vi "PRM1Z8_Init.vi"(8 "error in (no error)":errorcluster) -> (0 "error out":errorcluster, 3 "reference out":refnum<k24>)   [LabVIEW 2023, in "Thorlabs Polarizer.lvlib"]
uses:
  C:/FlashGordon/Development/dll/ThorLabs.MotionControl.KCube.DCServoCLI.dll
  dll/ThorLabs.MotionControl.KCube.DCServoCLI.dll
  C:/FlashGordon/Development/dll/Thorlabs.MotionControl.DeviceManagerCLI.dll
  dll/Thorlabs.MotionControl.DeviceManagerCLI.dll
  C:/FlashGordon/Development/dll/Thorlabs.MotionControl.GenericMotorCLI.dll
  dll/Thorlabs.MotionControl.GenericMotorCLI.dll
  Thorlabs Polarizer.lvlib
panel:
  out "Controller Information":T1
  out "Device list (serial no.)":string[](array[string])
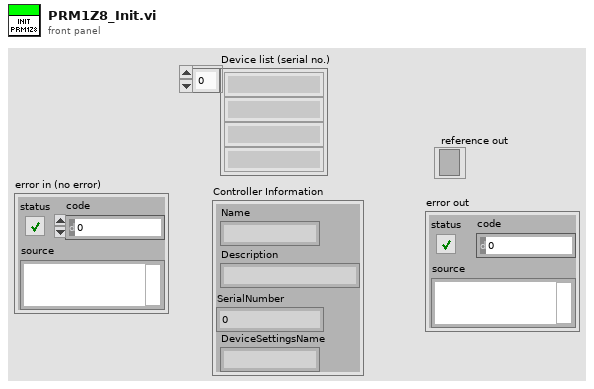
[diagram p1: front panel]
types:
  T1 = cluster{"Name":string, "Description":string, "SerialNumber":u32, "DeviceSettingsName":string}
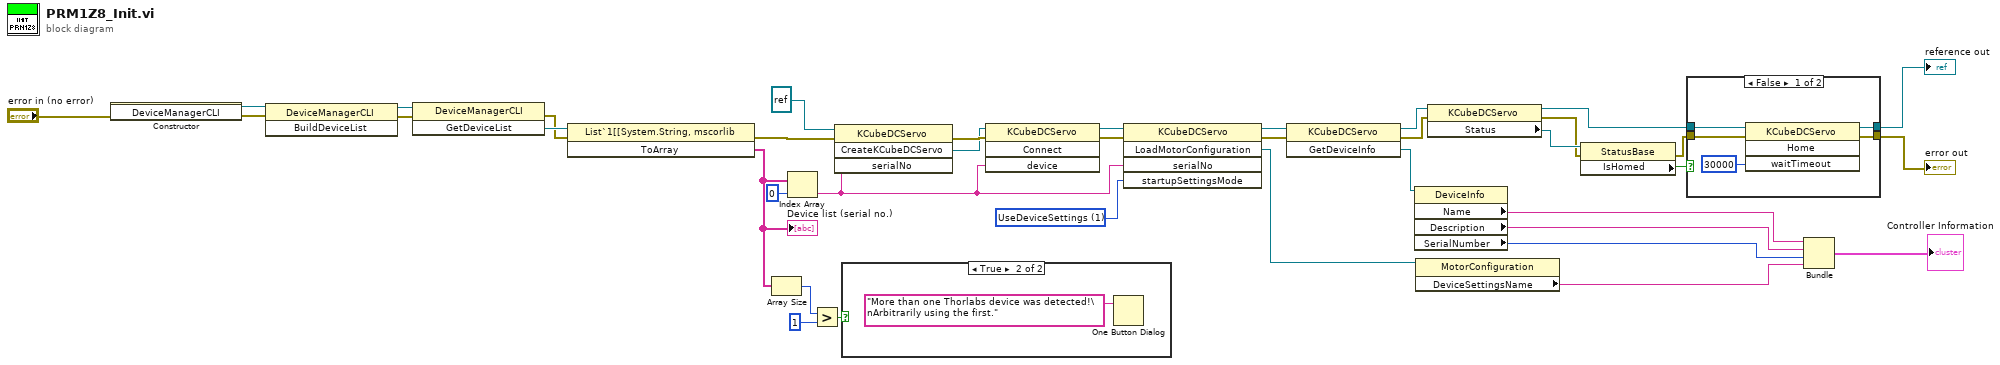
[diagram p0: block diagram]
diagram:
  w33 = 1 items=["UseDeviceSettings"=1, "UseFileSettings"=2, "UseConfiguredSettings"=3] ("startupSettingsMode")
  n1 = constructor class="DeviceManagerCLI"(error in="error in (no error)") -> (reference out=w15:refnum<k24>, error out=w16:errorcluster)  [unwired: 2 in, 1 out]
  n2 = invoke class="DeviceManagerCLI" method="BuildDeviceList"(reference=w15, error in=w16) -> (reference out=w28:refnum<k24>, error out=w30:errorcluster)  [unwired: 1 in, 1 out]
  n3 = invoke class="DeviceManagerCLI" method="GetDeviceList"(reference=w28, error in=w30) -> (error out=w27:errorcluster, "GetDeviceList"=w29:refnum<k24>)  [unwired: 1 in, 1 out]
  n4 = invoke class="List`1[[System.String, mscorlib" method="ToArray"(reference=w29, error in=w27) -> (error out=w26:errorcluster, "ToArray"=w14:string[])  [unwired: 1 in, 1 out]
  "Device list (serial no.)" <- w14
  n5 = Array Size(array=w14) -> (size(s)=w12:i32)
  n6 = Index Array(array=w14, index=0) -> (element=w24:string)
  n7 = Greater?(x=w12, y=1) -> (0:w13:bool)
  n8 = invoke class="KCubeDCServo" method="CreateKCubeDCServo"(reference=refnum<k24> refnum ("target class"), error in=w26, "serialNo"=w24) -> (error out=w35:errorcluster, "CreateKCubeDCServo"=w34:refnum<k24>)  [unwired: 1 in, 2 out]
  n9 = case shown="True" w13 {
    frame False {
    }
    frame True {
      n10 = One Button Dialog(message="More than one Thorlabs device was detected!\nArbitrarily using the first.") -> ()  [unwired: 1 in, 1 out]
    }
  }
  n11 = invoke class="KCubeDCServo" method="Connect"(reference=w34, error in=w35, "device"=w24) -> (reference out=w32:refnum<k24>, error out=w31:errorcluster)  [unwired: 1 in, 2 out]
  n12 = invoke class="KCubeDCServo" method="LoadMotorConfiguration"(reference=w32, error in=w31, "serialNo"=w24, "startupSettingsMode"=w33) -> (reference out=w8:refnum<k24>, error out=w18:errorcluster, "LoadMotorConfiguration"=w17:refnum<k24>)  [unwired: 1 in, 2 out]
  n13 = invoke class="KCubeDCServo" method="GetDeviceInfo"(reference=w8, error in=w18) -> (reference out=w2:refnum<k24>, error out=w5:errorcluster, "GetDeviceInfo"=w19:refnum<k24>)  [unwired: 1 in]
  n14 = property class="DeviceInfo"(reference=w19) -> ("Name"=w20:string, "Description"=w21:string, "SerialNumber"=w22:u32)  [unwired: 1 in, 2 out]
  n15 = property class="MotorConfiguration"(reference=w17) -> ("DeviceSettingsName"=w23:string)  [unwired: 1 in, 2 out]
  n16 = property class="KCubeDCServo"(reference=w2, error in=w5) -> (reference out=w1:refnum<k24>, error out=w4:errorcluster, "Status"=w7:refnum<k24>)
  n17 = property class="StatusBase"(reference=w7, error in=w4) -> (error out=w3:errorcluster, "IsHomed"=w6:bool)  [unwired: 1 out]
  n18 = case shown="False" w6 {
    tunnel: [w44 w46] -> w10
    tunnel: [w43 w45] -> w9
    tunnel: w1 -> [w41 w46]
    tunnel: w3 -> [w40 w45]
    frame False {
      n19 = invoke class="KCubeDCServo" method="Home"(reference=w41, error in=w40, "waitTimeout"=30000) -> (reference out=w44:refnum<k24>, error out=w43:errorcluster)  [unwired: 1 in, 2 out]
    }
    frame True {
    }
  }
  "reference out" <- w10
  "error out" <- w9
  n20 = Bundle("Name"=w20, "Description"=w21, "SerialNumber"=w22, "DeviceSettingsName"=w23) -> (→"Controller Information":T1)  [unwired: 1 in]
